vi "lvGS13.vi"() -> ()   [LabVIEW 2019]
uses:
  MoveSwitch.ctl
  <vilib>/Instr/_visa.llb/VISA Configure Serial Port (Instr).vi
panel:
  out "Version":string
  out "Local Origin":cluster{"X":dbl, "Y":dbl, "Z":dbl}
  out "Measure":bool
  out "Connecting to":string
  in  "Send G-code":bool
  out "Local-Pos":cluster{"X":dbl, "Y":dbl, "Z":dbl}
  out "M-Pos":cluster{"X":dbl, "Y":dbl, "Z":dbl}
  in  "Pos Button":bool
  out "Response":string
  in  "Local-Home":bool
  out "G-code list":string
  in  "Select G-code file":bool
  in  "One line Command":string
  out "MoveString":string
  in  "Manual Positioning":T1
  in  "distance(mm)":dbl=5.0
  in  "SetLocal":bool
  in  "Machine-Home":bool
  in  "Send":bool
  out "Command":string
  out "History":string
  in  "stop":bool
  in  "Grbl":refnum<visa-resource-name>="COM3"
  # "lv-G-Sender"
  # "計測・解析ラボ"
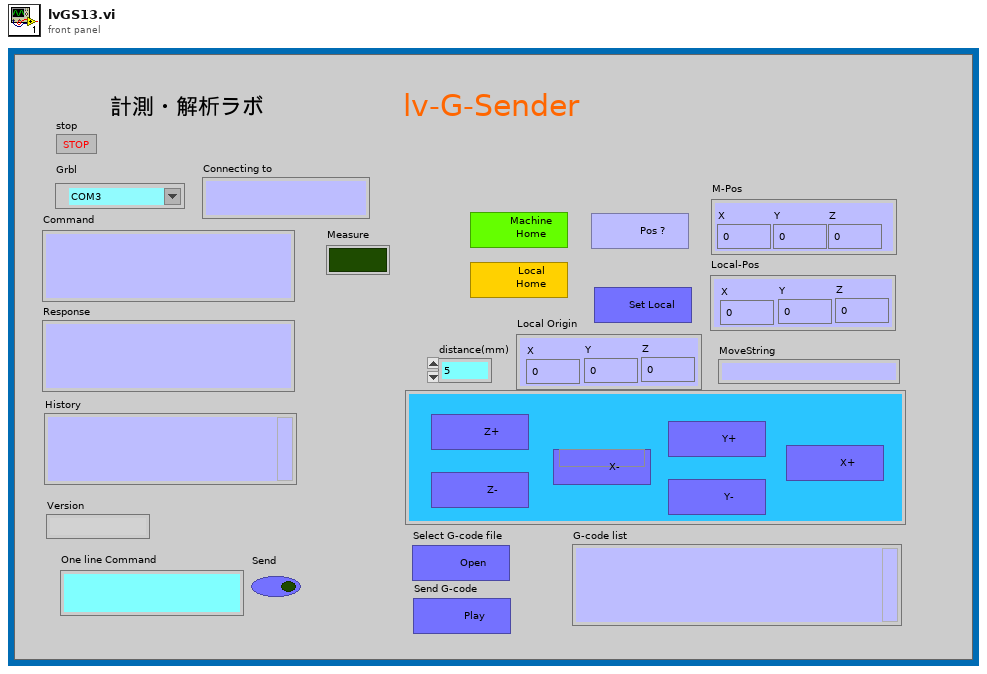
[diagram p1: front panel]
types:
  T1 = typedef "MoveSwitch.ctl" = cluster{"X+":bool, "X-":bool, "Y+":bool, "Y-":bool, "Z+":bool, "Z-":bool}
  T2 = cluster{"VISA resource name":refnum<visa-resource-name>, "baud rate":u32, "data bits":u16, "parity":u16, "stop bits":u16, "flow control":u16}
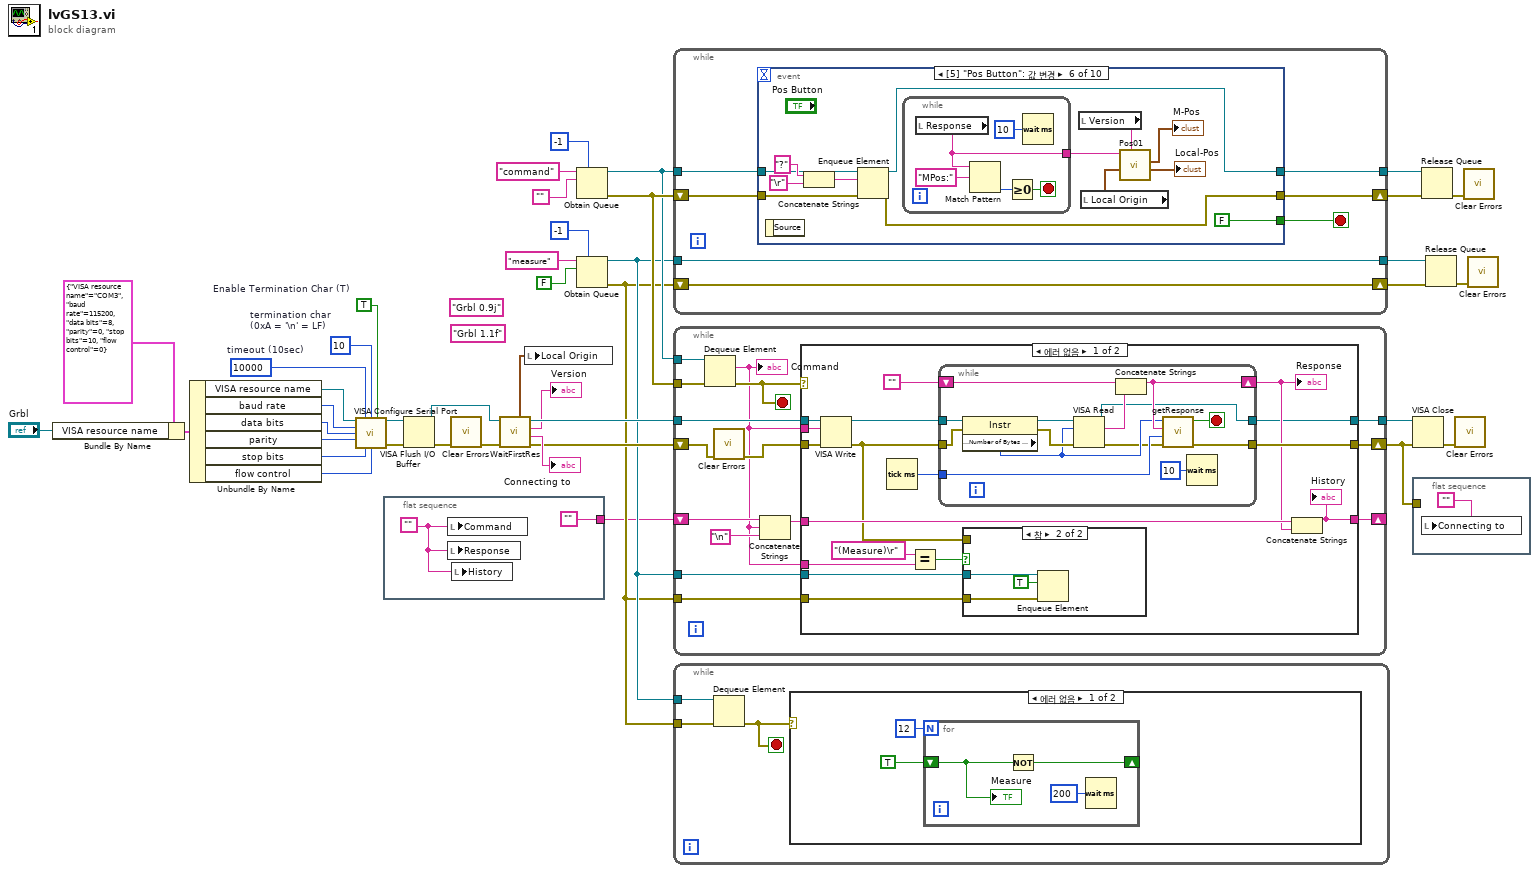
[diagram p0: block diagram]
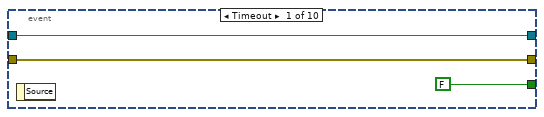
[diagram p3: hidden frame]
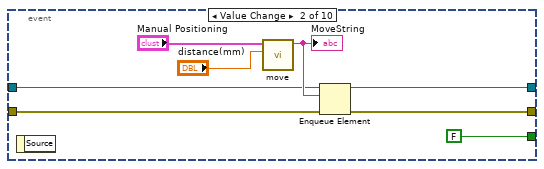
[diagram p4: hidden frame]
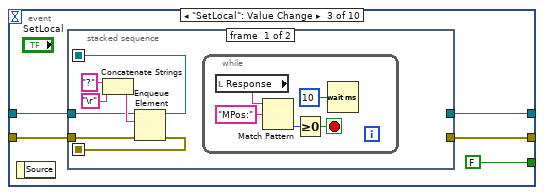
[diagram p5: hidden frame]
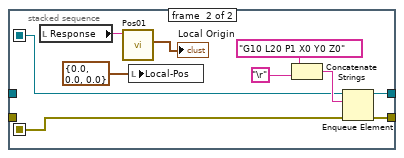
[diagram p6: hidden frame]
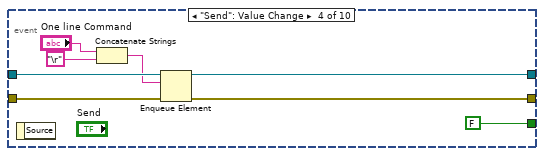
[diagram p7: hidden frame]
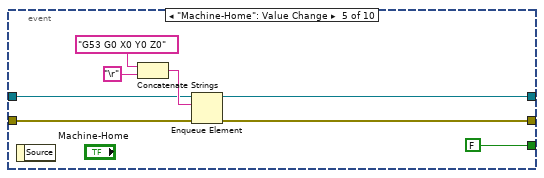
[diagram p8: hidden frame]
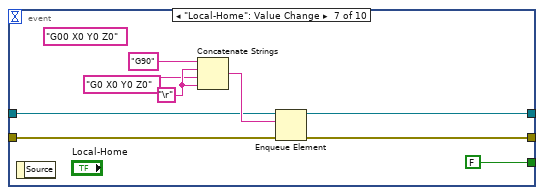
[diagram p9: hidden frame]
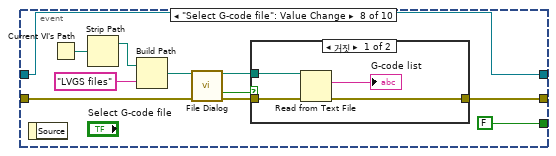
[diagram p10: hidden frame]
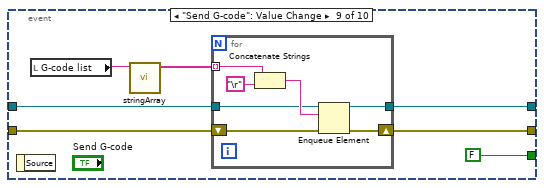
[diagram p12: hidden frame]
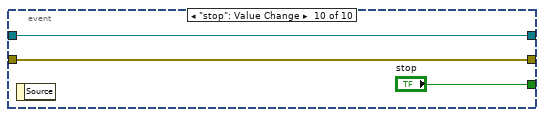
[diagram p13: hidden frame]
diagram:
  (unwired) "Grbl 1.1f" ("Version")
  (unwired) "Grbl 0.9j" ("Version")
  w20 = u8 10  # termination char (0xA = '\n' = LF)
  w31 = TRUE  # Enable Termination Char (T)
  w42 = u32 10000  # timeout (10sec)
  n1 = Bundle By Name(cluster=T2 {"VISA resource name"="COM3", "baud rate"=115200, "data bits"=8, "parity"=0, "stop bits"=10, "flow control"=0} ("COM"), "VISA resource name"="Grbl") -> (w38:T2)
  n2 = Unbundle By Name(w38) -> ("VISA resource name"=w37:refnum<visa-resource-name>, "baud rate"=w36:u32, "data bits"=w35:u16, "parity"=w34:u16, "stop bits"=w33:u16, "flow control"=w32:u16)
  n3 = call-poly "VISA Configure Serial Port"("VISA resource name"=w37, "timeout (10sec)"=w42, "termination char\n(0xA = '\\n' = LF)"=w20, "Enable Termination\nChar (T)"=w31, "baud rate (9600)"=w36, "data bits (8)"=w35, "parity (0:none)"=w34, "stop bits (10: 1 bit)"=w33, "flow control (0:none)"=w32) -> ("VISA resource name out"=w29:refnum<visa-resource-name>, "error out"=w30:errorcluster)  [unwired: 1 in, 4 out]
  n4 = flat-sequence {
    tunnel: [""] -> w3
    frame #0 {
      w44 = ""
      n5 = local write "Command"(w44) -> ()
      n6 = local write "Response"(w44) -> ()
      n7 = local write "History"(w44) -> ()
    }
  }
  n8 = VISA Flush I/O Buffer(VISA resource name=w29, error in (no error)=w30) -> (VISA resource name out=w19:refnum<visa-resource-name>, error out=w15:errorcluster)  [unwired: 1 in]
  n9 = call <vilib>:"Clear Errors.vi"("error in (no error)"=w15) -> ("error out"=w14:errorcluster)  [unwired: 5 in, 1 out]
  n10 = call "WaitFirstRes.vi"("error in (no error)"=w14, "VISA in"=w19) -> ("error out"=w13:errorcluster, "String"=→"Connecting to":string, "Version"=→"Version":string, "VISA out"=w18:refnum<visa-resource-name>, "Local Origin"=w1:cluster{"X":dbl, "Y":dbl, "Z":dbl})  [unwired: 4 in, 1 out]
  n11 = local write "Local Origin"(w1) -> ()
  n12 = Obtain Queue(max queue size (-1, unlimited)=-1, name (unnamed)="command", element data type="") -> (queue out=w16:refnum<queue>, error out=w21:errorcluster)  [unwired: 2 in, 1 out]
  n13 = Obtain Queue(max queue size (-1, unlimited)=-1, name (unnamed)="measure", element data type=FALSE) -> (queue out=w5:refnum<queue>, error out=w4:errorcluster)  [unwired: 2 in, 1 out]
  n14 = while {
    tunnel: w16 -> [w50]
    shift-right: [w48] -> w24
    shift-left: w21 -> [w49]
    tunnel: [w47] -> w23
    tunnel: [w46] -> w7
    tunnel: w5 -> [w46]
    shift-right: [w45] -> w6
    shift-left: w4 -> [w45]
    stop <- w51 stop-if-true
    n15 = event shown="[5] \"Pos Button\": 값 변경" {
      selector: _ -> [_ _ _ _ _ _ _ _ _ _]
      dyn-events: _ -> [_ _ _ _ _ _ _ _ _ _]
      timeout: _ -> [_ _ _ _ _ _ _ _ _ _]
      tunnel: [FALSE FALSE ("NewVal") FALSE ("stop") FALSE ("stop") FALSE ("stop") FALSE ("stop") FALSE ("stop") FALSE ("stop") FALSE ("stop") "stop"] -> w51
      tunnel: w50 -> [w52 w58 w64 w97 w98 w109 w128 w131 w152 w162]
      tunnel: w49 -> [w53 w57 w67 w96 w101 w112 w123 w132 w151 w161]
      tunnel: [w53 w56 w66 w90 w100 w107 w122 w134 w149 w161] -> w48
      tunnel: [w52 w55 w63 w91 w98 w109 w127 w131 w150 w162] -> w47
      event Timeout {
        n16 = event-data() -> ()  [unwired: 1 in, 1 out]
      }
      event Value Change {
        n17 = event-data() -> ()  [unwired: 1 in, 1 out]
        n18 = call "move.vi"("dist(mm)"="distance(mm)", "Manual Positioning"="Manual Positioning") -> ("MoveString"=w59:string)  [unwired: 9 in]
        "MoveString" <- w59
        n19 = Enqueue Element(queue=w58, element=w59, error in (no error)=w57) -> (queue out=w55:refnum<queue>, error out=w56:errorcluster)  [unwired: 1 in, 1 out]
      }
      event "SetLocal": Value Change {
        n20 = event-data() -> ()  [unwired: 1 in, 1 out]
        n21 = stacked-sequence {
          seq-local: [w69 _] -> [_ w83]
          seq-local: [w68 _] -> [_ w84]
          tunnel: w67 -> [w70 _]
          tunnel: [_ w85] -> w66
          tunnel: w64 -> [w71 _]
          tunnel: [_ w86] -> w63
          frame #0 {
            n22 = Concatenate Strings("?" ("Command 2"), "\r") -> (w72:string)
            n23 = Enqueue Element(queue=w71, element=w72, error in (no error)=w70) -> (queue out=w69:refnum<queue>, error out=w68:errorcluster)  [unwired: 1 in, 1 out]
            n24 = while {
              stop <- w77 stop-if-true
              n25 = local read "Response"() -> (w76:string)
              n26 = Match Pattern(string=w76, regular expression="MPos:") -> (offset past match=w78:i32)  [unwired: 1 in, 3 out]
              n27 = Greater Or Equal To 0?(x=w78) -> (x >= 0?=w77:bool)
              n28 = Wait (ms)(milliseconds to wait=u32 10) -> ()  [unwired: 1 out]
            }
          }
          frame #1 {
            n29 = local read "Response"() -> (w82:string)
            n30 = call "Pos01.vi"("String"=w82) -> ("M-Pos"=→"Local Origin":cluster{"X":dbl, "Y":dbl, "Z":dbl})  [unwired: 9 in, 1 out]
            n31 = local write "Local-Pos"(cluster{"X":dbl, "Y":dbl, "Z":dbl} {"X"=0.0, "Y"=0.0, "Z"=0.0} ("Local-Pos")) -> ()
            n32 = Concatenate Strings("G10 L20 P1 X0 Y0 Z0" ("format string"), "\r") -> (w88:string)
            n33 = Enqueue Element(queue=w83, element=w88, error in (no error)=w84) -> (queue out=w86:refnum<queue>, error out=w85:errorcluster)  [unwired: 1 in, 1 out]
          }
        }
      }
      event "Send": Value Change {
        n34 = event-data() -> ()  [unwired: 1 in, 1 out]
        n35 = Concatenate Strings("One line Command", "\r") -> (w92:string)
        n36 = Enqueue Element(queue=w97, element=w92, error in (no error)=w96) -> (queue out=w91:refnum<queue>, error out=w90:errorcluster)  [unwired: 1 in, 1 out]
      }
      event "Machine-Home": Value Change {
        n37 = event-data() -> ()  [unwired: 1 in, 1 out]
        n38 = Concatenate Strings("G53 G0 X0 Y0 Z0" ("Command 2"), "\r") -> (w102:string)
        n39 = Enqueue Element(queue=w98, element=w102, error in (no error)=w101) -> (error out=w100:errorcluster)  [unwired: 1 in, 2 out]
      }
      event "Pos Button": Value Change {
        n40 = event-data() -> ()  [unwired: 1 in, 1 out]
        n41 = Concatenate Strings("?" ("Command 2"), "\r") -> (w113:string)
        n42 = Enqueue Element(queue=w109, element=w113, error in (no error)=w112) -> (error out=w107:errorcluster)  [unwired: 1 in, 2 out]
        n43 = while {
          tunnel: [w117] -> w108
          stop <- w118 stop-if-true
          n44 = local read "Response"() -> (w117:string)
          n45 = Match Pattern(string=w117, regular expression="MPos:") -> (offset past match=w119:i32)  [unwired: 1 in, 3 out]
          n46 = Greater Or Equal To 0?(x=w119) -> (x >= 0?=w118:bool)
          n47 = Wait (ms)(milliseconds to wait=u32 10) -> ()  [unwired: 1 out]
        }
        n48 = local read "Version"() -> (w105:string)
        n49 = local read "Local Origin"() -> (w106:cluster{"X":dbl, "Y":dbl, "Z":dbl})
        n50 = call "Pos01.vi"("Version"=w105, "Local Origin"=w106, "String"=w108) -> ("W-Pos"=→"Local-Pos":cluster{"X":dbl, "Y":dbl, "Z":dbl}, "M-Pos"=→"M-Pos":cluster{"X":dbl, "Y":dbl, "Z":dbl})  [unwired: 7 in]
      }
      event "Local-Home": Value Change {
        (unwired) "G00 X0 Y0 Z0" ("Command 2")
        w126 = "\r"
        n51 = event-data() -> ()  [unwired: 1 in, 1 out]
        n52 = Concatenate Strings("G90" ("Command 2"), w126, "G0 X0 Y0 Z0" ("Command 2"), w126) -> (w129:string)
        n53 = Enqueue Element(queue=w128, element=w129, error in (no error)=w123) -> (queue out=w127:refnum<queue>, error out=w122:errorcluster)  [unwired: 1 in, 1 out]
      }
      event "Select G-code file": Value Change {
        n54 = event-data() -> ()  [unwired: 1 in, 1 out]
        n55 = Current VI's Path() -> (path=w141:path)
        n56 = Strip Path(path=w141) -> (stripped path=w140:path)  [unwired: 1 out]
        n57 = Build Path(base path=w140, name or relative path="LVGS files") -> (appended path=w138:path)
        n58 = call "File Dialog"("start path"=w138, "error in"=w132) -> ("selected path"=w136:path, "cancelled"=w137:bool, "error out"=w135:errorcluster)  [unwired: 10 in, 1 out]
        n59 = case shown="거짓" w137 {
          tunnel: w136 -> [w145 _]
          tunnel: w135 -> [w143 w146]
          tunnel: [w142 w146] -> w134
          frame False {
            n60 = Read from Text File(file (use dialog)=w145, error in=w143) -> (text=→"G-code list":string, error out=w142:errorcluster)  [unwired: 2 in, 2 out]
          }
          frame True {
          }
        }
      }
      event "Send G-code": Value Change {
        n61 = event-data() -> ()  [unwired: 1 in, 1 out]
        n62 = local read "G-code list"() -> (w153:string)
        n63 = call "stringArray.vi"("CNC strings"=w153) -> ("stringArray"=w148:string[])  [unwired: 10 in]
        n64 = for {
          tunnel: w152 -> [w158]
          tunnel: [w156] -> w150
          shift-right: [w155] -> w149
          shift-left: w151 -> [w157]
          tunnel: w148 -> [w154] mode=indexing
          n65 = Concatenate Strings(w154, "\r") -> (w159:string)
          n66 = Enqueue Element(queue=w158, element=w159, error in (no error)=w157) -> (queue out=w156:refnum<queue>, error out=w155:errorcluster)  [unwired: 1 in, 1 out]
        }
      }
      event "stop": Value Change {
        n67 = event-data() -> ()  [unwired: 1 in, 1 out]
      }
    }
  }
  n68 = while {
    tunnel: w18 -> [w177]
    shift-right: [w172] -> w12
    shift-left: w13 -> [w169]
    tunnel: [w173] -> w41
    shift-right: [w174] -> _
    shift-left: w3 -> [w176]
    tunnel: w16 -> [w178]
    tunnel: w21 -> [w171]
    tunnel: w5 -> [w165]
    tunnel: w4 -> [w164]
    stop <- w170 stop-if-true
    n69 = Dequeue Element(queue=w178, error in (no error)=w171) -> (element=w166:string, error out=w170:errorcluster)  [unwired: 1 in, 2 out]
    "Command" <- w166
    n70 = call <vilib>:"Clear Errors.vi"("error in (no error)"=w169) -> ("error out"=w168:errorcluster)  [unwired: 5 in, 1 out]
    n71 = Concatenate Strings(w176, w166, "\n") -> (w175:string)
    n72 = case shown="에러 없음" w170 {
      tunnel: w177 -> [w195 w214]
      tunnel: w166 -> [w193 _]
      tunnel: w175 -> [w190 w213]
      tunnel: [w189 w213] -> w174
      tunnel: [w179 w214] -> w173
      tunnel: [w192 w215] -> w172
      tunnel: w168 -> [w191 w215]
      tunnel: w166 -> [w180 _]
      tunnel: w165 -> [w183 _]
      tunnel: w164 -> [w182 _]
      frame No Error {
        n73 = VISA Write(VISA resource name=w195, write buffer=w193, error in (no error)=w191) -> (VISA resource name out=w194:refnum<visa-resource-name>, error out=w181:errorcluster)  [unwired: 1 out]
        n74 = Tick Count (ms)() -> (millisecond timer value=w186:u32)
        n75 = Equal?(x="(Measure)\r" ("y"), y=w180) -> (x = y?=w184:bool)
        n76 = while {
          tunnel: w194 -> [w212]
          tunnel: w181 -> [w200]
          shift-right: [w207] -> w187
          shift-left: "" -> [w209]
          tunnel: [w199] -> w179
          tunnel: [w202] -> w192
          tunnel: w186 -> [w206]
          stop <- w204 stop-if-true
          n77 = property class="Instr"(reference=w212, error in=w200) -> (reference out=w210:refnum<visa-resource-name>, error out=w211:errorcluster, "Serial Settings:Number of Bytes at Serial Port"=w205:u32)
          n78 = VISA Read(VISA resource name=w210, byte count=w205, error in (no error)=w211) -> (VISA resource name out=w199:refnum<visa-resource-name>, read buffer=w208:string, error out=w203:errorcluster)  [unwired: 1 out]
          n79 = Concatenate Strings(w209, w208) -> (w207:string)
          n80 = call "getResponse.vi"("error in (no error)"=w203, "ST"=w206, "string"=w207, "Bytes at Serial Port"=w205) -> ("error out"=w202:errorcluster, "done"=w204:bool)  [unwired: 5 in, 1 out]
          n81 = Wait (ms)(milliseconds to wait=u32 10) -> ()  [unwired: 1 out]
        }
        "Response" <- w187
        n82 = case shown="참" w184 {
          tunnel: w183 -> [_ w198]
          tunnel: w182 -> [_ w197]
          tunnel: w181 -> [_ _]
          frame False {
          }
          frame True {
            n83 = Enqueue Element(queue=w198, element=TRUE, error in (no error)=w197) -> ()  [unwired: 1 in, 3 out]
          }
        }
        n84 = Concatenate Strings(w190, w187) -> (w189:string)
        "History" <- w189
      }
      frame Error {
      }
    }
  }
  n85 = while {
    tunnel: w5 -> [w218]
    tunnel: w4 -> [w217]
    stop <- w216 stop-if-true
    n86 = Dequeue Element(queue=w218, error in (no error)=w217) -> (error out=w216:errorcluster)  [unwired: 1 in, 3 out]
    n87 = case shown="에러 없음" w216 {
      frame No Error {
        n88 = for {
          N: 12 -> [_]
          shift-right: [w222] -> _
          shift-left: TRUE ("OPERATION") -> [w223]
          n89 = Not(x=w223) -> (.not. x?=w222:bool)
          n90 = Wait (ms)(milliseconds to wait=u32 200) -> ()  [unwired: 1 out]
          "Measure" <- w223
        }
      }
      frame Error {
      }
    }
  }
  n91 = VISA Close(VISA resource name=w41, error in (no error)=w12) -> (error out=w28:errorcluster)
  n92 = flat-sequence {
    tunnel: w12 -> [_]
    frame #0 {
      n93 = local write "Connecting to"("") -> ()
    }
  }
  n94 = Release Queue(queue=w23, error in (no error)=w24) -> (error out=w22:errorcluster)  [unwired: 1 in, 2 out]
  n95 = Release Queue(queue=w7, error in (no error)=w6) -> (error out=w8:errorcluster)  [unwired: 1 in, 2 out]
  n96 = call <vilib>:"Clear Errors.vi"("error in (no error)"=w28) -> ()  [unwired: 5 in, 2 out]
  n97 = call <vilib>:"Clear Errors.vi"("error in (no error)"=w22) -> ()  [unwired: 5 in, 2 out]
  n98 = call <vilib>:"Clear Errors.vi"("error in (no error)"=w8) -> ()  [unwired: 5 in, 2 out]
